vi "CD Storage Library Loader.vi"   [LabVIEW 2019]
uses:
  Library/Custom Devices Storage.lvlib
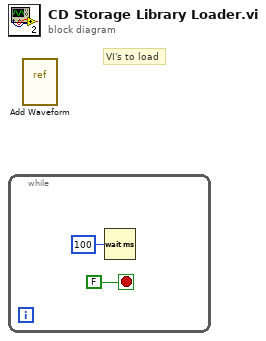
[diagram p0: block diagram]
diagram:
  # "VI's to load"
  n1 = while {
    stop <- FALSE stop-if-true
    n2 = Wait (ms)(milliseconds to wait=u32 100) -> ()  [unwired: 1 out]
  }
  n3 = vi-ref "Add Waveform.vi"() -> ()  [unwired: 1 out]
